vi "generate FE.vi"(5 "doubleFace?":bool=TRUE, 6 "stepsize":dbl=0.1, 7 "Mode":enum16{"FR", "FC"}(ring), 10 "Zmag":dbl[](array[numeric]), 11 "Z":dbl[](array[numeric])) -> (2 "XYͼ":cluster{dbl[], dbl[]}(graph))   [LabVIEW 2017]
uses:
  <vilib>/Analysis/baseanly.llb/Mean (DBL).vi
  <vilib>/Analysis/NI_AALBase.lvlib
panel:
  in  "A":dbl=102.7
  in  "B":dbl=-1.184
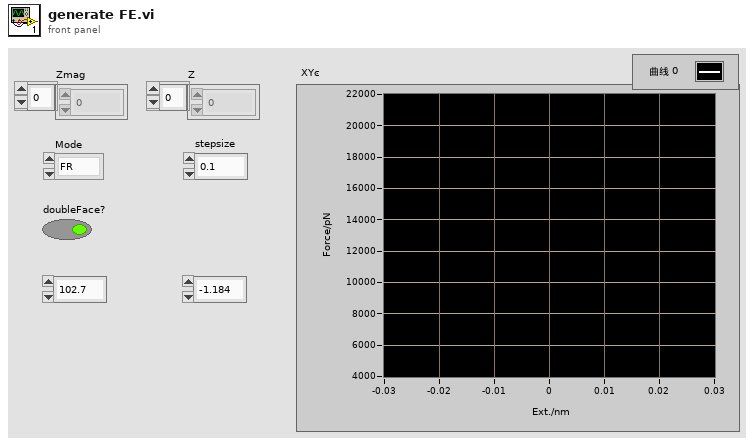
[diagram p1: front panel]
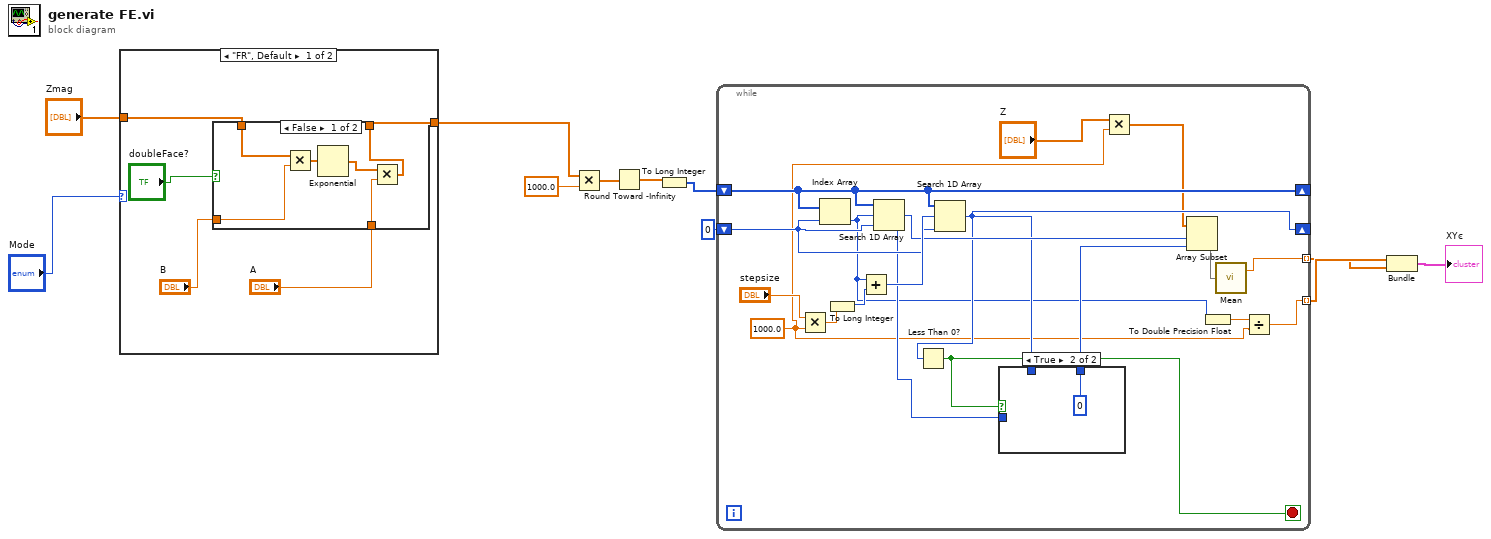
[diagram p0: block diagram]
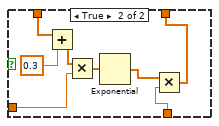
[diagram p2: hidden frame]
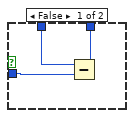
[diagram p4: hidden frame]
diagram:
  n1 = case shown="\"FR\", Default" "Mode" {
    tunnel: "Zmag" -> [w13 w31]
    tunnel: [w12 w31] -> w7
    frame "FR", Default {
      n2 = case shown="False" "doubleFace?" {
        tunnel: w13 -> [w22 w25]
        tunnel: [w19 w23] -> w12
        tunnel: "B" -> [w18 w28]
        tunnel: "A" -> [w17 w27]
        frame False {
          n3 = Multiply(x=w22, y=w18) -> (x*y=w21:dbl[])
          n4 = Exponential(1:w21) -> (0:w20:dbl[])
          n5 = Multiply(x=w20, y=w17) -> (x*y=w19:dbl[])
        }
        frame True {
          n6 = Add(x=w25, y=0.3) -> (x+y=w26:dbl[])
          n7 = Multiply(x=w26, y=w28) -> (x*y=w30:dbl[])
          n8 = Exponential(1:w30) -> (0:w29:dbl[])
          n9 = Multiply(x=w29, y=w27) -> (x*y=w23:dbl[])
        }
      }
    }
    frame "FC" {
    }
  }
  n10 = Multiply(x=w7, y=1000.0) -> (x*y=w5:dbl[])
  n11 = Round Toward -Infinity(1:w5) -> (0:w4:dbl[])
  n12 = To Long Integer(number=w4) -> (32bit integer=w3:i32[])
  n13 = while {
    shift-right: [w45] -> _
    shift-left: w3 -> [w45]
    shift-right: [w42] -> _
    shift-left: 0 ("index") -> [w48]
    tunnel: [w46] -> w1 mode=indexing
    tunnel: [w32] -> w2 mode=indexing
    stop <- w44 stop-if-true
    w34 = 1000.0
    n14 = Multiply(x="stepsize", y=w34) -> (x*y=w39:dbl)
    n15 = Index Array(array=w45, index=w48) -> (element=w35:i32)
    n16 = To Long Integer(number=w39) -> (32bit integer=w38:i32)
    n17 = Add(x=w35, y=w38) -> (x+y=w49:i32)
    n18 = Search 1D Array(1D array=w45, element=w35, start index (0)=w48) -> (index of element=w43:i32)
    n19 = Search 1D Array(1D array=w45, element=w49, start index (0)=w48) -> (index of element=w42:i32)
    n20 = Less Than 0?(x=w42) -> (x < 0?=w44:bool)
    n21 = case shown="True" w44 {
      tunnel: w43 -> [w52 _]
      tunnel: w42 -> [w51 _]
      tunnel: [w50 0] -> w41
      frame False {
        n22 = Subtract(x=w51, y=w52) -> (x-y=w50:i32)
      }
      frame True {
      }
    }
    n23 = Multiply(x="Z", y=w34) -> (x*y=w36:dbl[])
    n24 = Array Subset(array=w36, index=w43, length=w41) -> (w47:dbl[])
    n25 = To Double Precision Float(number=w35) -> (double precision float=w33:dbl)
    n26 = call-poly <vilib>:"Mean.vi"("X"=w47) -> ("mean"=w46:dbl)  [unwired: 1 out]
    n27 = Divide(x=w33, y=w34) -> (x/y=w32:dbl)
  }
  n28 = Bundle(w2, w1) -> (→"XYͼ":cluster{dbl[], dbl[]})  [unwired: 1 in]
